vi "Set Value.vi"(8 "error in (no error)":errorcluster, 10 "Value":i64, 11 "SnailNum in":refnum<class "SnailNum.lvclass">) -> (0 "error out":errorcluster, 3 "SnailNum out":refnum<class "SnailNum.lvclass">)   [LabVIEW 2020, in "SnailNum.lvclass"]
uses:
  SnailNum.lvclass
  SnailNum.lvclass/SnailNum.ctl
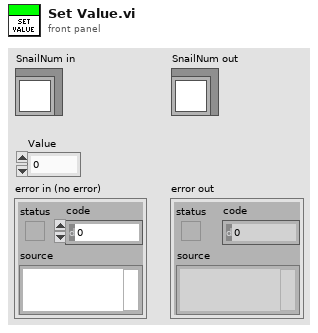
[diagram p1: front panel]
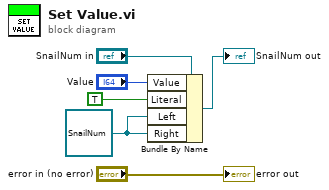
[diagram p0: block diagram]
diagram:
  w1 = refnum<class "SnailNum.lvclass"> refnum ("SnailNum.lvclass")
  n1 = Bundle By Name(cluster="SnailNum in", "Value"="Value", "Literal"=TRUE, "Left"=w1, "Right"=w1) -> (→"SnailNum out":refnum<class "SnailNum.lvclass">)
  "error out" <- "error in (no error)"
